vi "variable.vi"() -> ()   [LabVIEW 2020]
panel:
  out "A":i32
  in  "stop":bool
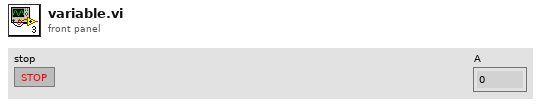
[diagram p1: front panel]
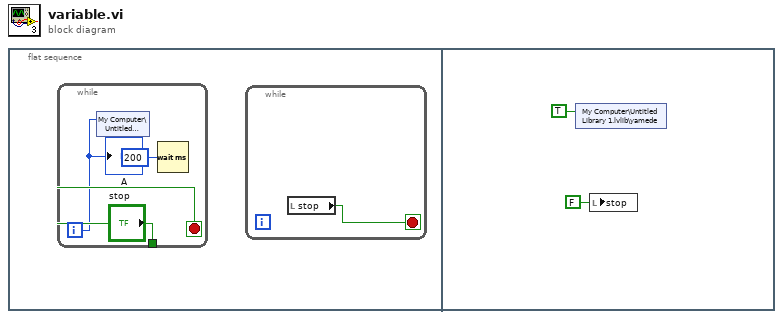
[diagram p0: block diagram]
diagram:
  n1 = flat-sequence {
    frame #0 {
      n2 = while {
        tunnel: ["stop"] -> _
        i -> [w3]
        stop <- "stop" stop-if-true
        n3 = shared-variable "My Computer\\Untitled Library 1.lvlib\\A"(w3) -> ()  [unwired: 1 in, 1 out]
        n4 = Wait (ms)(milliseconds to wait=u32 200) -> ()  [unwired: 1 out]
        "A" <- w3
      }
      n5 = while {
        stop <- w1 stop-if-true
        n6 = local read "stop"() -> (w1:bool)
      }
    }
    frame #1 {
      n7 = shared-variable "My Computer\\Untitled Library 1.lvlib\\yamede"(TRUE ("yamede")) -> ()  [unwired: 1 in, 1 out]
      n8 = local write "stop"(FALSE ("stop")) -> ()
    }
  }
